vi "attribute_write_none.vi"(5 "Repeated Capability":string, 7 "Attribute":T1={"Identifier"="", "Descriptive name"="", "Data Type"=enum."Integer 32", "Command"="", "Access"=2, "Range Table"="", "Read Callback"="", "Write Callback"="", "Range Callback"="", "Check Callback"="", "Rngtable Callback"="", "Coerce Callback"="", "Supported Models"="", "Instrument Options"="", "Repeated Capabilities"="", "Check Status Callback"="", "Index"=0, "Flag: OPC Wait"=FALSE, "Flag: Dont check status"=FALSE, "Flag: Cache Only"=FALSE} {"Access" items=["Read Only", "Write Only", "Read/Write"]}, 8 "error in":errorcluster, 11 "VISA resource name":refnum<visa-resource-name>) -> (0 "error out":errorcluster, 3 "VISA resource name out":refnum<visa-resource-name>)   [LabVIEW 2014, in "rszvl_rsidr_core.lvlib"]
uses:
  rszvl_rsidr_core.lvlib
  type_Attribute.ctl
  type_Attribute_Data_Type.ctl
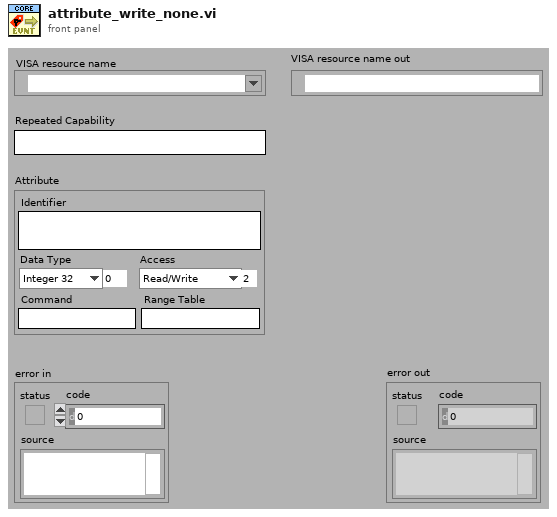
[diagram p1: front panel]
types:
  T1 = typedef "rszvl_rsidr_core.lvlib/type_Attribute.ctl" = cluster{"Identifier":string, "Descriptive name":string, "Data Type":T2, "Command":string, "Access":u16, "Range Table":string, "Read Callback":string, "Write Callback":string, "Range Callback":string, "Check Callback":string, "Rngtable Callback":string, "Coerce Callback":string, "Supported Models":string, "Instrument Options":string, "Repeated Capabilities":string, "Check Status Callback":string, "Index":i32, "Flag: OPC Wait":bool, "Flag: Dont check status":bool, "Flag: Cache Only":bool}
  T2 = typedef "rszvl_rsidr_core.lvlib/type_Attribute_Data_Type.ctl" = enum16{"Integer 32", "Double", "String", "Boolean", "None", "Integer 64"}
  T3 = typedef "rszvl_rsidr_core.lvlib/type_Session_Data.ctl" = cluster{"Instr type":string, "Instr type for err. msg.":string, "Installed Options":string[], "OPC Timeout":i32, "Query Instrument Status":bool, "Check Range":bool, "Check Options":bool, "Add LF to Write":bool, "Simulate":bool, "Logging":bool, "Logging params":variant, "Interface Type":enum16{"Unknown", "GPIB", "VXI", "GPIB_VXI", "ASRL", "PXI", "TCPIP", "USB", "SOCKET"}, "Fast Sweep":i32, "AdditionalFlags":i32, "WaitBeforeWrite":i32, "WaitBeforeRead":i32, "BinDataChunkSize":i64}
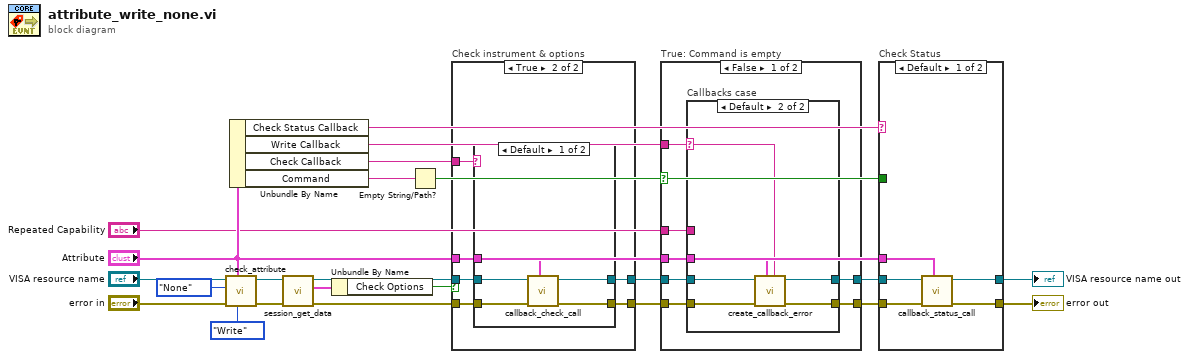
[diagram p0: block diagram]
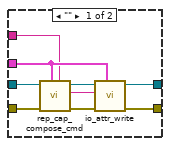
[diagram p2: hidden frame]
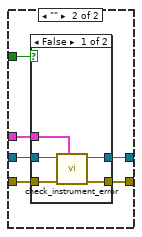
[diagram p4: hidden frame]
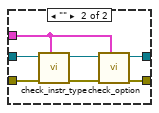
[diagram p7: hidden frame]
diagram:
  n1 = call "check_attribute.vi"("Access"=enum16{"Read", "Write"}."Write", "Attribute"="Attribute", "error in"="error in", "Data Type"=type_Attribute_Data_Type."None", "VISA resource name"="VISA resource name") -> ("error out"=w11:errorcluster, "VISA resource name out"=w12:refnum<visa-resource-name>)  [unwired: 5 in]
  n2 = Unbundle By Name("Attribute") -> ("Check Status Callback"=w3:string, "Write Callback"=w13:string, "Check Callback"=w14:string, "Command"=w1:string)
  n3 = call "session_get_data.vi"("error in"=w11, "VISA resource name"=w12) -> ("error out"=w9:errorcluster, "Session User Data out"=w7:T3, "VISA resource name out"=w10:refnum<visa-resource-name>)  [unwired: 7 in]
  n4 = Unbundle By Name(w7) -> ("Check Options"=w8:bool)
  n5 = Empty String/Path?(string/path=w1) -> (empty?=w23:bool)
  n6 = case "Check instrument & options" shown="True" w8 {
    tunnel: [w25 w31] -> w5
    tunnel: [w24 w30] -> w4
    tunnel: "Attribute" -> [_ w29]
    tunnel: w14 -> [_ w28]
    tunnel: w10 -> [w25 w27]
    tunnel: w9 -> [w24 w26]
    frame False {
    }
    frame True {
      n7 = case shown="Default" w28 {
        tunnel: [w35 w41] -> w31
        tunnel: [w33 w40] -> w30
        tunnel: w26 -> [w34 w39]
        tunnel: w29 -> [w32 w37]
        tunnel: w27 -> [w36 w38]
        frame Default {
          n8 = call "callback_check_call.vi"("Attribute"=w32, "error in"=w34, "VISA resource name"=w36) -> ("error out"=w33:errorcluster, "VISA resource name out"=w35:refnum<visa-resource-name>)  [unwired: 7 in]
        }
        frame "" {
          n9 = call "check_instr_type.vi"("Attribute"=w37, "error in"=w39, "VISA resource name"=w38) -> ("error out"=w43:errorcluster, "VISA resource name out"=w42:refnum<visa-resource-name>)  [unwired: 6 in, 1 out]
          n10 = call "check_option.vi"("Attribute"=w37, "error in"=w43, "VISA resource name"=w42) -> ("error out"=w40:errorcluster, "VISA resource name out"=w41:refnum<visa-resource-name>)  [unwired: 7 in]
        }
      }
    }
  }
  n11 = case "True: Command is empty" shown="False" w23 {
    tunnel: "Repeated Capability" -> [w50 _]
    tunnel: w4 -> [w49 w66]
    tunnel: w5 -> [w48 w67]
    tunnel: "Attribute" -> [w47 _]
    tunnel: [w46 w67] -> w16
    tunnel: [w45 w66] -> w15
    tunnel: w13 -> [w44 _]
    frame False {
      n12 = case "Callbacks case" shown="Default" w44 {
        selector: w44 -> [_ w60]
        tunnel: w48 -> [w58 w64]
        tunnel: w49 -> [w56 w65]
        tunnel: w50 -> [w51 _]
        tunnel: [w55 w62] -> w46
        tunnel: [w54 w63] -> w45
        tunnel: w47 -> [w52 w61]
        frame "" {
          n13 = call "rep_cap_compose_cmd.vi"("Repeated Capability"=w51, "Attribute"=w52, "error in"=w56, "VISA resource name"=w58) -> ("error out"=w57:errorcluster, "Command out"=w53:string, "VISA resource name out"=w59:refnum<visa-resource-name>)  [unwired: 5 in]
          n14 = call "io_attr_write.vi"("Attribute"=w52, "error in"=w57, "write buffer"=w53, "VISA resource name"=w59) -> ("error out"=w54:errorcluster, "VISA resource name out"=w55:refnum<visa-resource-name>)  [unwired: 6 in]
        }
        frame Default {
          n15 = call "create_callback_error.vi"("Callback Name"=w60, "Attribute"=w61, "error in"=w65, "VISA resource name"=w64) -> ("error out"=w63:errorcluster, "VISA resource name out"=w62:refnum<visa-resource-name>)  [unwired: 6 in]
        }
      }
    }
    frame True {
    }
  }
  n16 = case "Check Status" shown="Default" w3 {
    tunnel: w15 -> [w72 w77]
    tunnel: [w71 w76] -> w22
    tunnel: [w70 w75] -> w21
    tunnel: w16 -> [w69 w78]
    tunnel: "Attribute" -> [w68 w74]
    tunnel: w23 -> [_ w73]
    frame Default {
      n17 = call "callback_status_call.vi"("Attribute"=w68, "error in"=w72, "VISA resource name"=w69) -> ("error out"=w71:errorcluster, "VISA resource name out"=w70:refnum<visa-resource-name>)  [unwired: 7 in]
    }
    frame "" {
      n18 = case shown="False" w73 {
        tunnel: w78 -> [w83 w85]
        tunnel: w77 -> [w82 w84]
        tunnel: [w81 w84] -> w76
        tunnel: [w80 w85] -> w75
        tunnel: w74 -> [w79 _]
        frame False {
          n19 = call "check_instrument_error.vi"("Attribute"=w79, "error in"=w82, "VISA resource name"=w83) -> ("error out"=w81:errorcluster, "VISA resource name out"=w80:refnum<visa-resource-name>)  [unwired: 7 in]
        }
        frame True {
        }
      }
    }
  }
  "error out" <- w22
  "VISA resource name out" <- w21
